vi "Add Poll.vi"(8 "error in (no error)":errorcluster, 11 "Node Ptr":u64 format="%.0x") -> (0 "error out":errorcluster)   [LabVIEW 2019, in "Diagnostics Addon System Explorer.lvlib"]
uses:
  Diagnostics Addon System Explorer.lvlib
  Types/Poll.LinkedNode.ctl
  Types/FG.Action.ctl
  Types/Poll.Create.ctl
  Types/Poll.Settings.ctl
  Shared/Types/DPID.Rate.ctl
  Shared/Types/Type.ctl
  Shared/SubVIs/Constants.vi
  Shared/Diagnostics Addon Shared.lvlib
  <vilib>/NI VeriStand/Custom Device API/Custom Device API.lvlib
  <vilib>/NI VeriStand/Custom Device Tools/Custom Device Utility Library/Custom Device Utility Library.lvlib
panel:
  in  "Tag":string
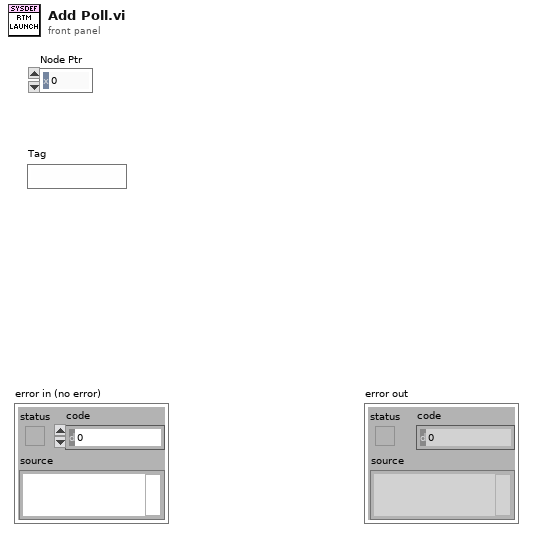
[diagram p1: front panel]
types:
  T1 = typedef "Diagnostics Addon System Explorer.lvlib/Poll.LinkedNode.ctl" = cluster{"Node ID":u64}
  T2 = typedef "Custom Device API.lvlib/Custom Device Item Ref.ctl" = u64
  T3 = typedef "Diagnostics Addon System Explorer.lvlib/FG.Action.ctl" = enum16{"Get", "Set"}
  T4 = typedef "Diagnostics Addon System Explorer.lvlib/Poll.Settings.ctl" = cluster{"Input Channels":T1[], "Speed":T5}
  T5 = typedef "Diagnostics Addon Shared.lvlib/DPID.Rate.ctl" = enum16{"Slow", "Medium", "Fast"}
  T6 = typedef "Custom Device API.lvlib/Custom Device Item Info.ctl" = cluster{"Name":string, "Is Channel":bool, "GUID":string, "Is Waveform":bool}
  T7 = typedef "Diagnostics Addon Shared.lvlib/Type.ctl" = enum16{"DID", "CDID", "PID", "CPID", "Read Memory", "Write Memory", "IO Control", "Routine Start", "Routine Request", "Routine Stop", "User Defined", "DTC Control", "Clear DTCs", "Read DTCs", "Start DTCs", "DTC Change Count", "Tester Present", "Unlock ECU", "Reset ECU", "Diag Session Control", "Communication Control", "DPID Control", "Poll Control", "Diag CAN Control"}
  T8 = typedef "Diagnostics Addon System Explorer.lvlib/Poll.Create.ctl" = cluster{"Name":string, "Settings":T4}
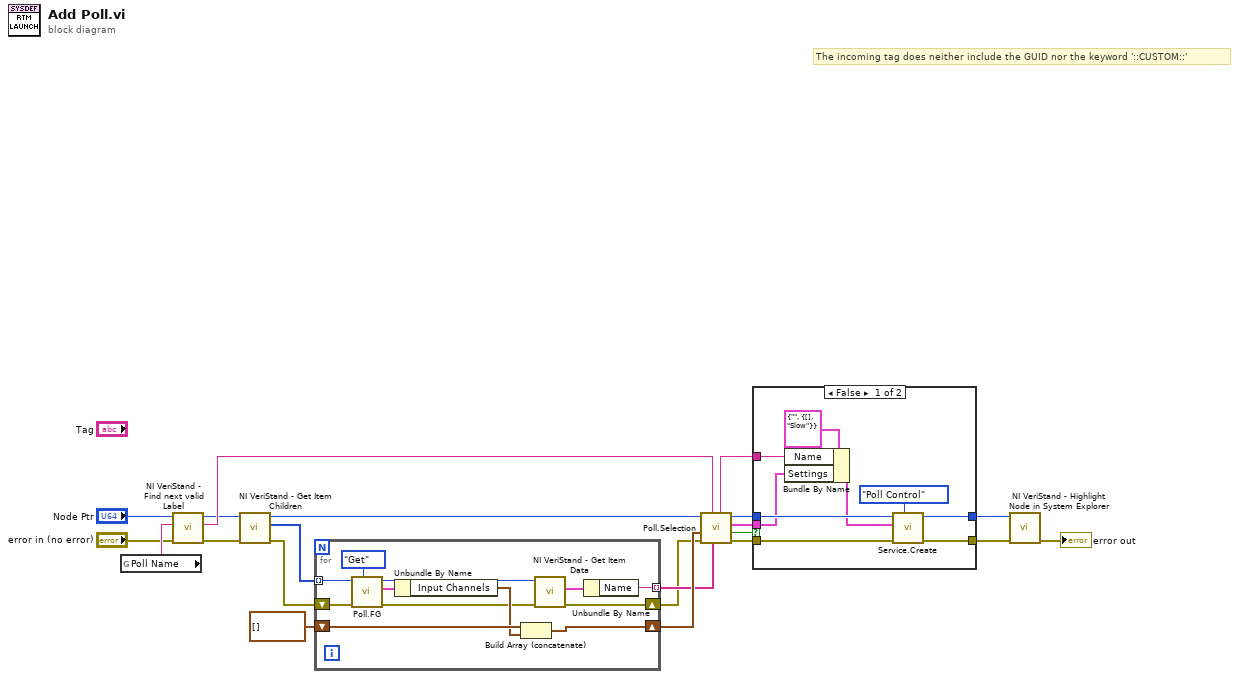
[diagram p0: block diagram]
diagram:
  # "The incoming tag does neither include the GUID nor the keyword '::CUSTOM::'"
  n1 = global read "Constants.vi" "Poll Name"() -> (w21:string)
  n2 = call <vilib>:"NI VeriStand - Find next valid Label.vi"("error in (no error)"="error in (no error)", "Label"=w21, "Item Ref in"="Node Ptr") -> ("error out"=w5:errorcluster, "Label out"=w10:string, "Item Ref out"=w4:T2)  [unwired: 4 in, 2 out]
  n3 = call <vilib>:"NI VeriStand - Get Item Children.vi"("error in (no error)"=w5, "Item Ref in"=w4) -> ("error out"=w17:errorcluster, "Child Refs"=w3:T2[], "Item Ref out"=w2:T2)  [unwired: 6 in, 1 out]
  n4 = for {
    tunnel: w3 -> [w31] mode=indexing
    shift-right: [w25] -> w7
    shift-left: w17 -> [w30]
    shift-right: [w27] -> w15
    shift-left: T1[] [] ("Input Channels") -> [w29]
    tunnel: [w22] -> w13 mode=indexing
    n5 = call "Poll.FG.vi"("Action"=FG.Action."Get", "error in"=w30, "Parent Ref"=w31) -> ("error out"=w26:errorcluster, "Selected Channels out"=w33:T4, "Parent Ref Out"=w24:T2)  [unwired: 6 in]
    n6 = Unbundle By Name(w33) -> ("Input Channels"=w28:T1[])
    n7 = Build Array (concatenate)(w29, w28) -> (w27:T1[])
    n8 = call <vilib>:"NI VeriStand - Get Item Data.vi"("error in (no error)"=w26, "Item Ref in"=w24) -> ("error out"=w25:errorcluster, "Item Info"=w23:T6)  [unwired: 6 in, 2 out]
    n9 = Unbundle By Name(w23) -> ("Name"=w22:string)
  }
  n10 = call "Poll.Selection.vi"("Existing Names"=w13, "Name"=w10, "error in (no error)"=w7, "Already Used"=w15, "Node Ptr"=w2) -> ("error out"=w20:errorcluster, "Cancel out"=w12:bool, "Selected Channels"=w14:T4, "Node Ptr out"=w1:T2, "Name out"=w11:string)  [unwired: 2 in]
  n11 = case shown="False" w12 {
    tunnel: w20 -> [w42 w44]
    tunnel: w1 -> [w41 w43]
    tunnel: [w40 w44] -> w19
    tunnel: [w39 w43] -> w18
    tunnel: w14 -> [w35 _]
    tunnel: w11 -> [w36 _]
    frame False {
      n12 = Bundle By Name(cluster=T8 {"Name"="", "Settings"={"Input Channels"=[], "Speed"=enum."Slow"}} ("output cluster"), "Name"=w36, "Settings"=w35) -> (w34:T8)
      n13 = call "Service.Create.vi"("Type"=Type."Poll Control", "error in (no error)"=w42, "Variant"=w34, "Section Ptr"=w41) -> ("error out"=w40:errorcluster, "Parent Ref out"=w39:T2)  [unwired: 6 in]
    }
    frame True {
    }
  }
  n14 = call <vilib>:"NI VeriStand - Highlight Node in System Explorer.vi"("error in (no error)"=w19, "Item Ref in"=w18) -> ("error out"=→"error out":errorcluster)  [unwired: 8 in, 1 out]
